vi "GetThingNames.vi"() -> (2 "Comm":T1, 3 "Things":string[](array[string]))   [LabVIEW 2020]
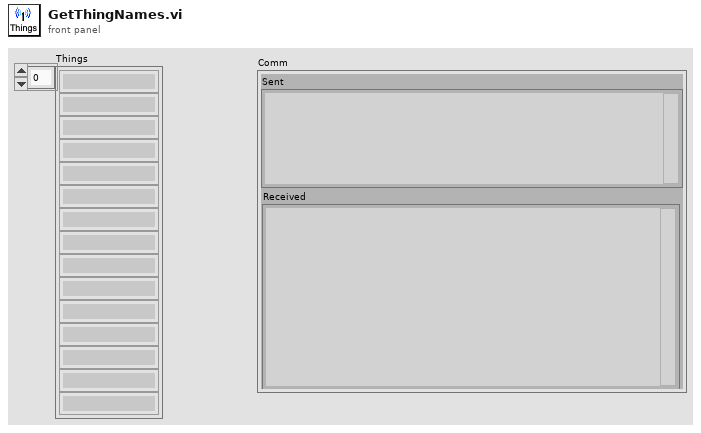
[diagram p1: front panel]
types:
  T1 = cluster{"url":string, "sent headers":string, "sent body":string, "headers":string, "body":string, "Sent":string, "Received":string}
  T2 = enum16{"GET", "PUT", "POST", "MultiPOST", "DELETE"}
  T3 = cluster{"rows":cluster{"avatar":string, "name":string, "description":string, "homeMashup":string, "isSystemObject":bool}[]}
  T4 = cluster{"Name":string, "BaseURL":string, "AppKey":string, "Headers":string[], "Timeout":i32}
  T5 = cluster{"avatar":string, "name":string, "description":string, "homeMashup":string, "isSystemObject":bool}[]
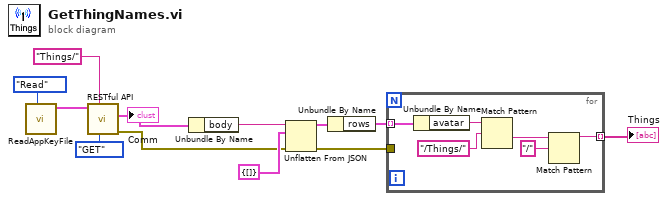
[diagram p0: block diagram]
diagram:
  n1 = call "ReadAppKeyFile.vi"("Task"=enum16{"Read", "Write"}."Read") -> ("Device Out"=w11:T4)  [unwired: 8 in, 2 out]
  n2 = call "RESTful API.vi"("Method"=T2."GET", "url"="Things/", "Device In"=w11) -> ("error out"=w2:errorcluster, "Comm"=w10:T1)  [unwired: 6 in, 1 out]
  "Comm" <- w10
  n3 = Unbundle By Name(w10) -> ("body"=w6:string)
  n4 = Unflatten From JSON(JSON string=w6, type and defaults=T3 {"rows"=[]}, error in (no error)=w2) -> (value=w8:T3, error out=w1:errorcluster)  [unwired: 4 in]
  n5 = Unbundle By Name(w8) -> ("rows"=w9:T5)
  n6 = for {
    tunnel: w9 -> [w18] mode=indexing
    tunnel: [w13] -> w12 mode=indexing
    tunnel: w1 -> [_]
    n7 = Unbundle By Name(w18) -> ("avatar"=w17:string)
    n8 = Match Pattern(string=w17, regular expression="/Things/") -> (after substring=w15:string)  [unwired: 1 in, 3 out]
    n9 = Match Pattern(string=w15, regular expression="/") -> (before substring=w13:string)  [unwired: 1 in, 3 out]
  }
  "Things" <- w12
